vi "WaitReady.vi"(2 "PortNumber":i32, 3 "Residence time in ms":i32=1) -> (0 "OK Done":bool, 1 "String Received":string)   [LabVIEW 2015]
panel:
  # "Port Number 0=COM1"
  # "Send '!:\\r\\n' and wait for 'R\\r\\n'.\nAn Error occurs when timed out."
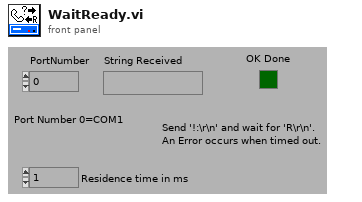
[diagram p1: front panel]
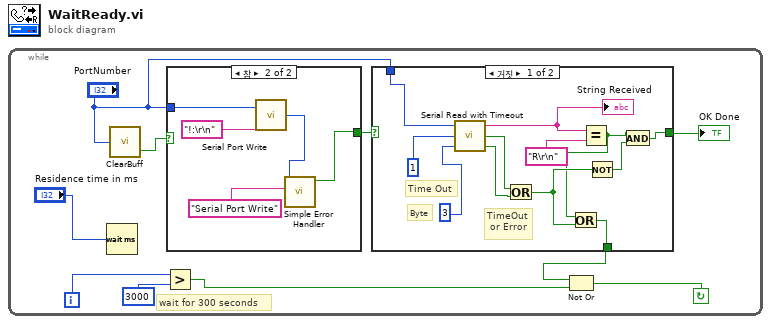
[diagram p0: block diagram]
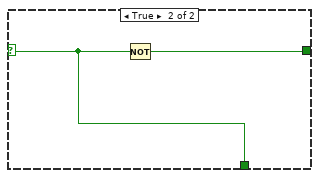
[diagram p2: hidden frame]
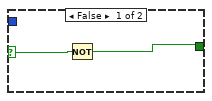
[diagram p3: hidden frame]
diagram:
  n1 = while {
    i -> [w8]
    stop <- w5 continue-if-true
    # "wait for 300 seconds"
    n2 = Wait (ms)(milliseconds to wait="Residence time in ms") -> ()  [unwired: 1 out]
    n3 = call "ClearBuff.vi"("PortNumber"="PortNumber") -> ("OK Done"=w2:bool)  [unwired: 1 out]
    n4 = Greater?(x=w8, y=3000) -> (0:w6:bool)
    n5 = case shown="참" w2 {
      selector: w2 -> [w26 _]
      tunnel: "PortNumber" -> [_ w30]
      tunnel: [w25 w27] -> w10
      frame False {
        n6 = Not(x=w26) -> (.not. x?=w25:bool)
      }
      frame True {
        n7 = call <vilib>:"Serial Port Write.vi"("string to write"="!:\r\n", "port number"=w30) -> ("error code"=w28:i32)
        n8 = call <vilib>:"Simple Error Handler.vi"("error code (no error:0)"=w28, "error source (\" \")"="Serial Port Write") -> ("error?"=w27:bool)  [unwired: 2 in, 5 out]
      }
    }
    n9 = case shown="거짓" w10 {
      selector: w10 -> [_ w23]
      tunnel: "PortNumber" -> [w20 _]
      tunnel: [w17 w23] -> w7
      tunnel: [w12 w24] -> w4
      frame False {
        # "TimeOut\n or Error"
        # "Byte"
        # "Time Out"
        n10 = call "Serial Read with Timeout.vi"("Bytes to Read"=3, "Timeout Limit"=1, "Port Number"=w20) -> ("Error Out"=w18:bool, "Timeout"=w19:bool, "Serial Read"=w16:string)
        "String Received" <- w16
        n11 = Or(x=w19, y=w18) -> (x .or. y?=w13:bool)
        n12 = Equal?(x=w16, y="R\r\n") -> (x = y?=w11:bool)
        n13 = Or(x=w11, y=w13) -> (x .or. y?=w17:bool)
        n14 = Not(x=w13) -> (.not. x?=w14:bool)
        n15 = And(x=w11, y=w14) -> (x .and. y?=w12:bool)
      }
      frame True {
        n16 = Not(x=w23) -> (.not. x?=w24:bool)
      }
    }
    "OK Done" <- w4
    n17 = Not Or(1:w6, 2:w7) -> (0:w5:bool)
  }
